vi "Run Test.vi"(8 "error in (no error)":errorcluster, 11 "Example Test In":refnum<class "Example Test.lvclass">) -> (0 "error out":errorcluster, 1 "Positions":i32[](array[numeric]), 2 "Tests Passed":bool[](array[boolean]), 3 "Example Test Out":refnum<class "Example Test.lvclass">, 5 "Fail Codes":string[](array[string]))   [LabVIEW 2017, in "Example Test.lvclass"]
uses:
  Example Test.lvclass
  C:/Test System Services/Acrobat Framework/CBTF Modules/Tests/Test Class/Test Class.lvclass
  Classes/Application/Class/Application.lvclass
  Test Class/Test Class.lvclass
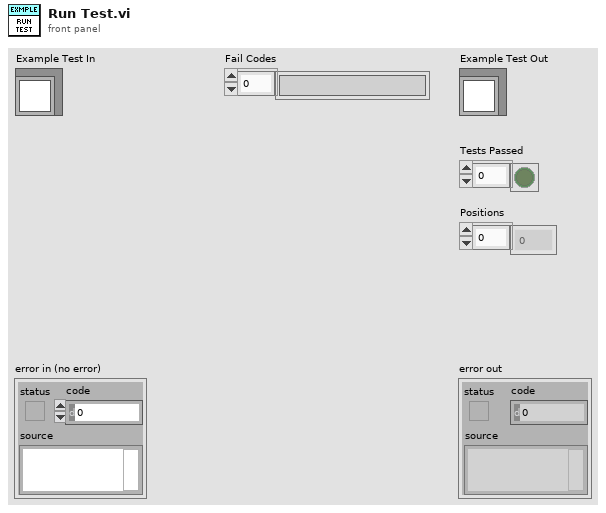
[diagram p1: front panel]
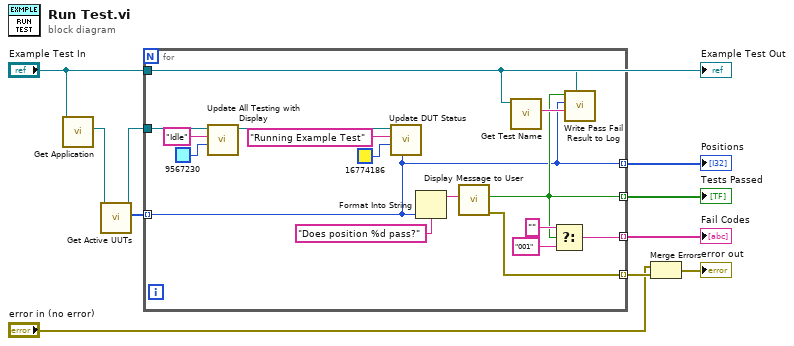
[diagram p0: block diagram]
diagram:
  n1 = call "Get Application.vi"("Test Class in"="Example Test In") -> ("Application.lvlib:Application.lvclass"=w6:refnum<class "Application.lvclass">)  [unwired: 9 in, 1 out]
  n2 = call "Get Active UUTs.vi"("Application in"=w6) -> ("Active Positions"=w4:u32[], "Application out"=w5:refnum<class "Application.lvclass">)  [unwired: 8 in, 1 out]
  n3 = for {
    tunnel: [w23] -> w10 mode=indexing
    tunnel: w5 -> [w26]
    tunnel: [w12] -> w9 mode=indexing
    tunnel: w4 -> [w11] mode=indexing
    tunnel: [w11] -> w3 mode=indexing
    tunnel: [w15] -> w2 mode=indexing
    tunnel: "Example Test In" -> [w13]
    n4 = call "Update All Testing with Display.vi"("BG Color"=u32 9567230, "Message ('')"="Idle", "Application in"=w26) -> ("Application out"=w18:refnum<class "Application.lvclass">)  [unwired: 7 in, 1 out]
    n5 = call "Update DUT Status.vi"("Position"=w11, "BG Color"=u32 16774186, "Message ('')"="Running Example Test", "Application in"=w18) -> ()  [unwired: 6 in, 2 out]
    n6 = Format Into String(format string="Does position %d pass?" ("Message"), w11) -> (resulting string=w21:string)  [unwired: 2 in, 1 out]
    n7 = call "Display Message to User"("Message"=w21) -> ("error out"=w23:errorcluster, "OK"=w12:bool)  [unwired: 9 in]
    n8 = call "Get Test Name.vi"("Test Class in"=w13) -> ("Test Name"=w14:string)  [unwired: 9 in, 1 out]
    n9 = Select(t="", s=w12, f="001") -> (s? t:f=w15:string)
    n10 = call "Write Pass Fail Result to Log.vi"("Test Class in"=w13, "Label"=w14, "Position"=w11, "Result"=w12) -> ()  [unwired: 7 in, 1 out]
  }
  "Tests Passed" <- w9
  "Fail Codes" <- w2
  "Positions" <- w3
  n11 = Merge Errors("error in (no error)", w10) -> (→"error out":errorcluster)
  "Example Test Out" <- "Example Test In"
